vi "[subVI]_unflatten_and_plot.vi"(11 "S300 data":string) -> (3 "XY Graph":cluster{"X":dbl, "Y":dbl}[](graph))   [LabVIEW 2013]
panel:
  # "Input"
  # "Output"
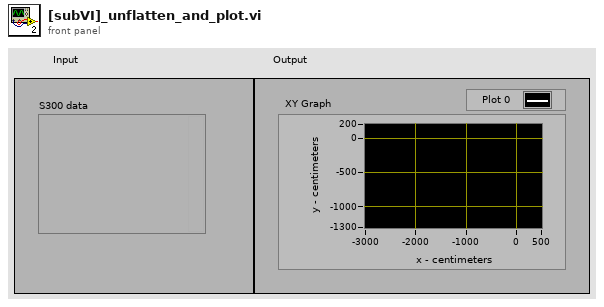
[diagram p1: front panel]
types:
  T1 = enum16{"big-endian, network order", "native, host order", "little-endian"}
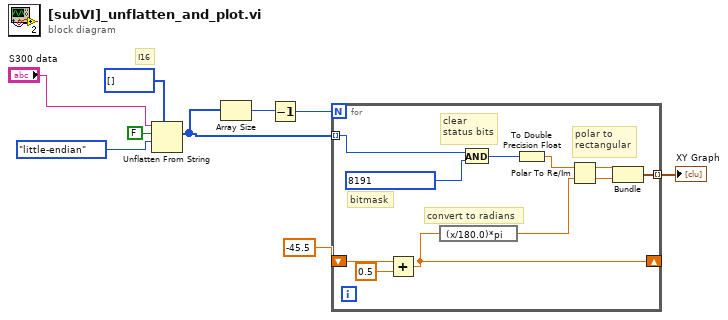
[diagram p0: block diagram]
diagram:
  # "I16"
  n1 = Unflatten From String(type=i16[] [], binary string="S300 data", data includes array or string size? (T)=FALSE, byte order (0:big-endian, network order)=T1."little-endian") -> (value=w3:i16[])  [unwired: 1 in, 2 out]
  n2 = Array Size(array=w3) -> (size(s)=w5:i32)
  n3 = Decrement(x=w5) -> (x-1=w4:i32)
  n4 = for {
    N: w4 -> [_]
    tunnel: w3 -> [w19] mode=indexing
    shift-right: [w15] -> _
    shift-left: -45.5 -> [w17]
    tunnel: [w10] -> w1 mode=indexing
    # "polar to\nrectangular"
    # "convert to radians"
    # "clear \nstatus bits"
    # "bitmask"
    n5 = Add(x=w17, y=0.5) -> (x+y=w15:dbl)
    n6 = expression code="(x/180.0)*pi" ("degrees to radians")(w15) -> (w14:dbl)
    n7 = And(x=w19, y=i16 8191) -> (x .and. y?=w16:i16)
    n8 = To Double Precision Float(number=w16) -> (double precision float=w13:dbl)
    n9 = Polar To Re/Im(2:w14, 3:w13) -> (0:w11:dbl, 1:w12:dbl)
    n10 = Bundle(w12, w11) -> (w10:cluster{dbl, dbl})  [unwired: 1 in]
  }
  "XY Graph" <- w1
